vi "Read Dual Fan Actor.vi"(11 "硬件蒸发冷却器":refnum<class "HW Evaporative Cooler.lvclass">) -> (2 "双风扇":refnum<class "Dual Fan.lvclass">)   [LabVIEW 2013, in "HW Evaporative Cooler.lvclass"]
uses:
  HW Evaporative Cooler.lvclass
  Dual Fan/Dual Fan/Dual Fan.lvclass
  HW Dual Fan/HW Dual Fan.lvclass
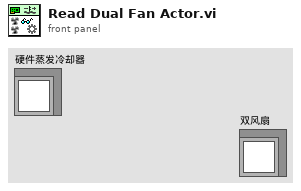
[diagram p1: front panel]
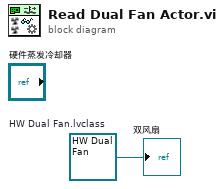
[diagram p0: block diagram]
diagram:
  w1 = refnum<class "HW Dual Fan.lvclass"> refnum  # HW Dual Fan.lvclass
  "双风扇" <- w1
